vi "HeaterDialog.vi"(8 "Error In":errorcluster, 11 "Heater Configuration In":T1={"VISA Resource"="", "COM Port"=1, "Setpoint"=0.0, "Standby?"=FALSE}) -> (0 "Error Out":errorcluster, 2 "Cancelled?":bool, 3 "Heater Configuration Out":T1={"VISA Resource"="", "COM Port"=1, "Setpoint"=0.0, "Standby?"=FALSE})   [LabVIEW 2012]
uses:
  HeaterConfiguration.ctl
  libs/LV-Utilities/LV-Utilities.lvlib
panel:
  in  "COM Port":u8=1
  in  "Heater State":enum16{"Run", "Standby"}(ring)
  in  "CANCEL":bool
  in  "DONE":bool
  in  "Setpoint (C)":dbl=nan format="%.1f"
  # "COM Port"
  # "PID State"
  # "Temperature (C)"
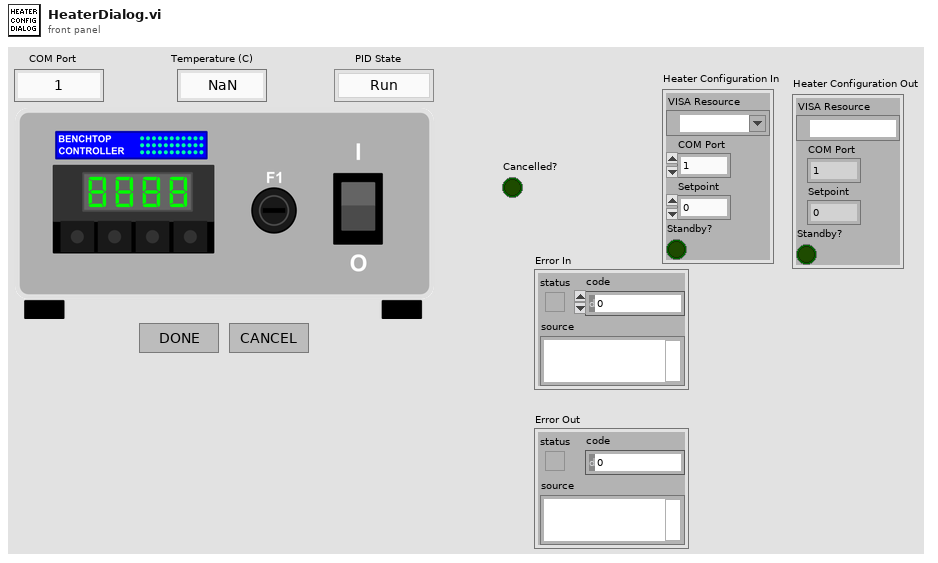
[diagram p1: front panel]
types:
  T1 = typedef "HeaterConfiguration.ctl" = cluster{"VISA Resource":refnum<visa-resource-name>, "COM Port":u8, "Setpoint":dbl, "Standby?":bool}
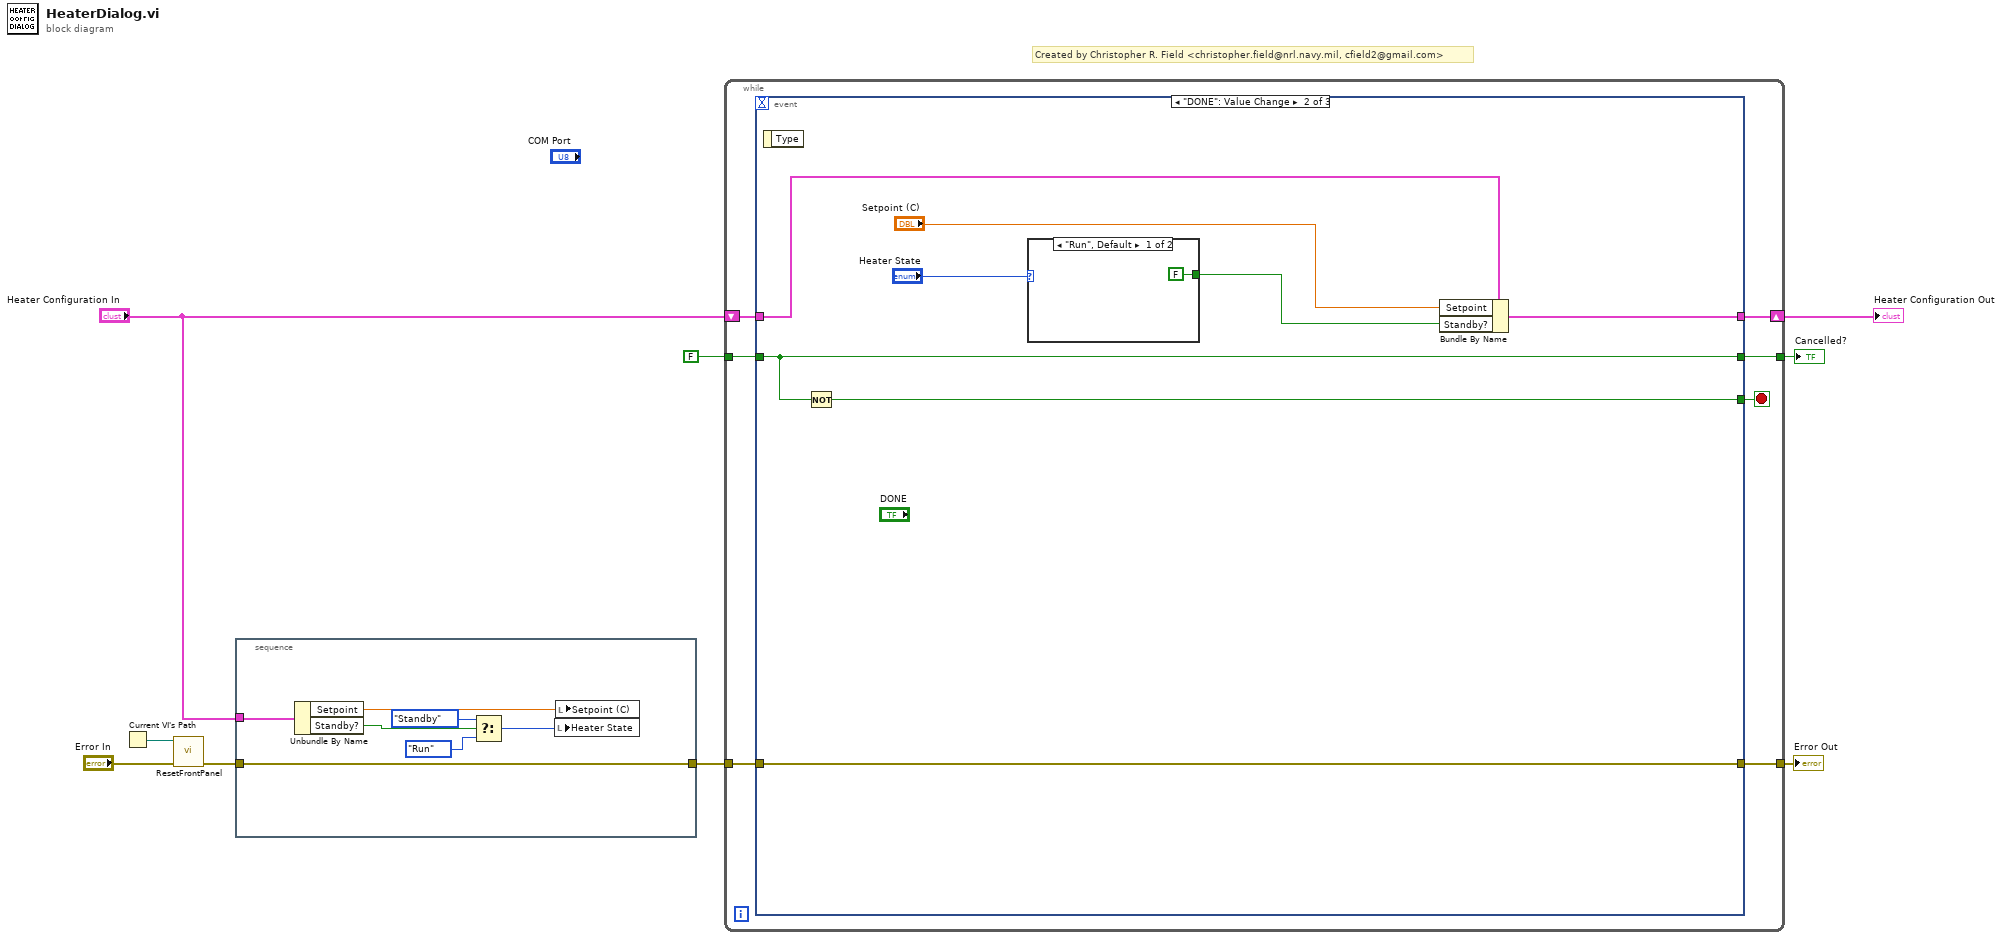
[diagram p0: block diagram]
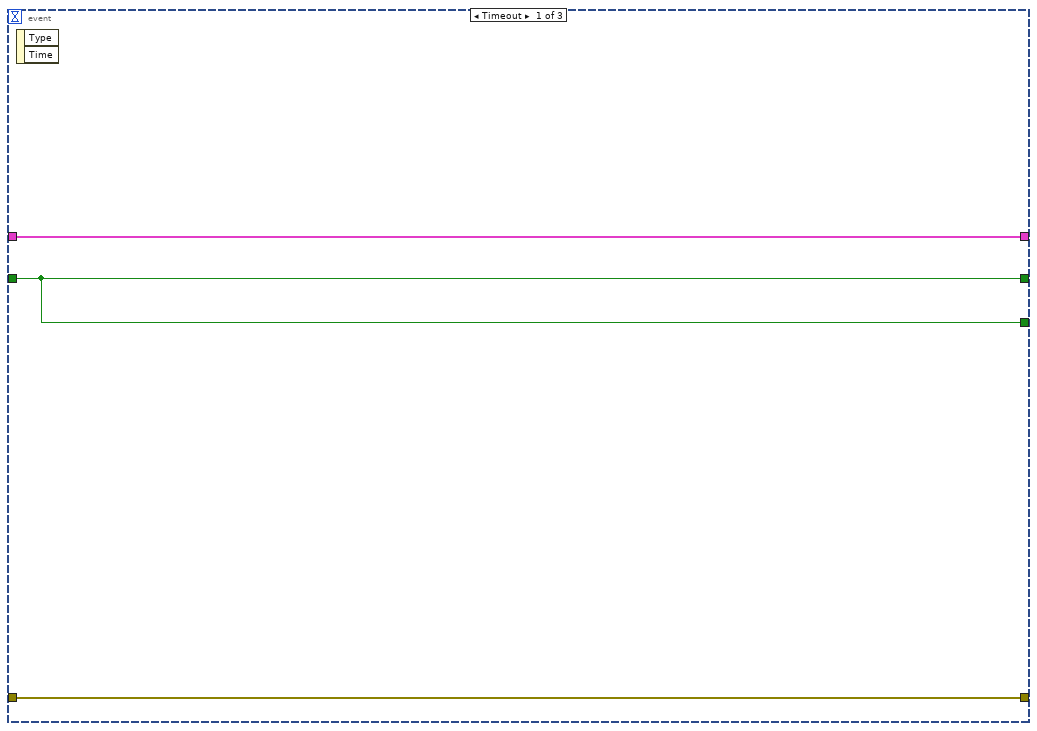
[diagram p2: hidden frame]
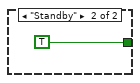
[diagram p3: hidden frame]
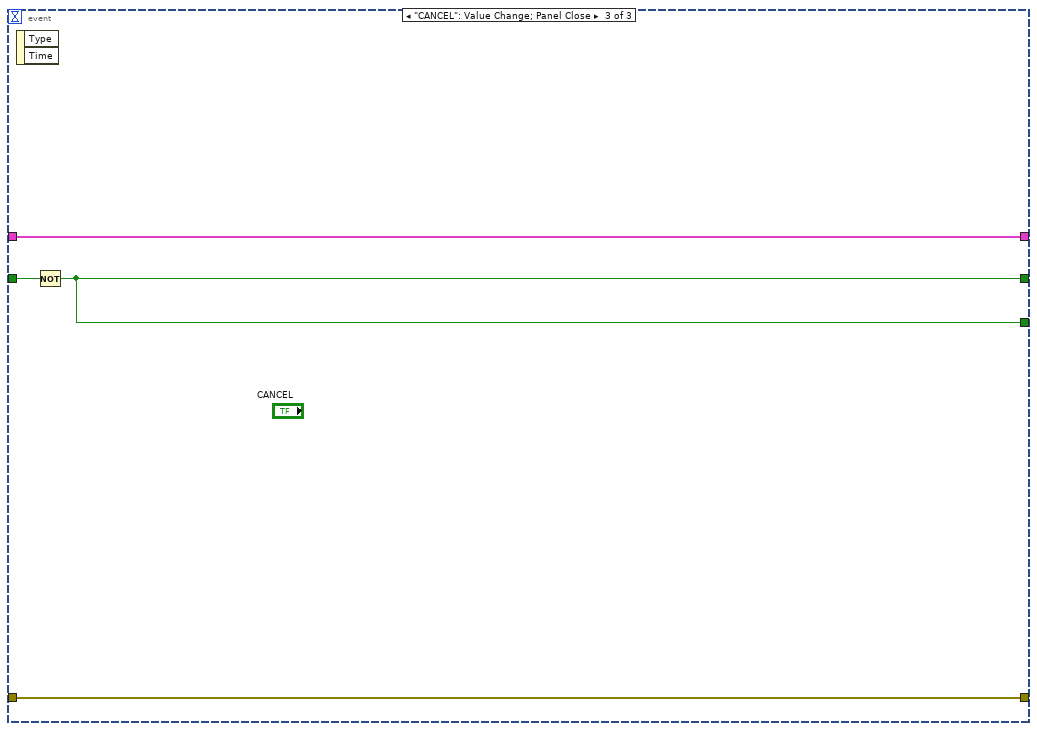
[diagram p4: hidden frame]
diagram:
  # "Created by Christopher R. Field <christopher.field@nrl.navy.mil, cfield2@gmail.com>"
  n1 = Current VI's Path() -> (path=w6:path)
  n2 = call "ResetFrontPanel.vi"("Error In"="Error In", "VI Path"=w6) -> ("Error Out"=w4:errorcluster)  [unwired: 9 in]
  n3 = stacked-sequence {
    tunnel: w4 -> [w15]
    tunnel: [w15] -> w3
    tunnel: "Heater Configuration In" -> [w10]
    frame #0 {
      n4 = Unbundle By Name(w10) -> ("Setpoint"=w16:dbl, "Standby?"=w14:bool)
      n5 = Select(t=enum16{"Run", "Standby"}."Standby", s=w14, f=enum16{"Run", "Standby"}."Run" ("Heater State In")) -> (s? t:f=w12:enum16{"Run", "Standby"})
      n6 = local write "Heater State"(w12) -> ()
      n7 = local write "Setpoint (C)"(w16) -> ()
    }
  }
  n8 = while {
    tunnel: FALSE -> [w23]
    tunnel: [w21] -> w8
    tunnel: w3 -> [w20]
    tunnel: [w19] -> w7
    shift-right: [w17] -> w1
    shift-left: "Heater Configuration In" -> [w18]
    stop <- w22 stop-if-true
    n9 = event shown="[1] \"DONE\": Value Change" {
      selector: _ -> [_ _ _]
      dyn-events: _ -> [_ _ _]
      timeout: _ -> [_ _ _]
      tunnel: w23 -> [w26 w33 w40]
      tunnel: [w26 w34 w39] -> w22
      tunnel: [w26 w33 w39] -> w21
      tunnel: w20 -> [w25 w32 w38]
      tunnel: [w25 w32 w38] -> w19
      tunnel: w18 -> [w24 w28 w37]
      tunnel: [w24 w27 w37] -> w17
      event Timeout {
        n10 = event-data() -> ()  [unwired: 1 in, 2 out]
      }
      event "DONE": Value Change {
        n11 = event-data() -> ()  [unwired: 1 in, 1 out]
        n12 = Not(x=w33) -> (.not. x?=w34:bool)
        n13 = case shown="\"Run\", Default" "Heater State" {
          tunnel: [FALSE TRUE] -> w29
          frame "Run", Default {
          }
          frame "Standby" {
          }
        }
        n14 = Bundle By Name(cluster=w28, "Setpoint"="Setpoint (C)", "Standby?"=w29) -> (w27:T1)
      }
      event "CANCEL": Value Change; Panel Close {
        n15 = event-data() -> ()  [unwired: 1 in, 2 out]
        n16 = Not(x=w40) -> (.not. x?=w39:bool)
      }
    }
  }
  "Cancelled?" <- w8
  "Error Out" <- w7
  "Heater Configuration Out" <- w1
